vi "Apply Motor Transfer.vi"(10 "Right Motor":dbl, 11 "Left Motor":dbl) -> (2 "Right Motor Voltage":dbl, 3 "Left Motor Voltage":dbl)   [LabVIEW 2016]
uses:
  Globals/Motor Transfer.vi
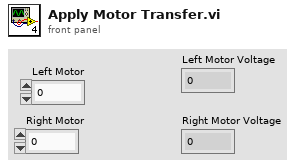
[diagram p1: front panel]
types:
  T1 = cluster{"Positive":cluster{"Slope":dbl, "Intercept":dbl}, "Negative":cluster{"Slope":dbl, "Intercept":dbl}}[]
  T2 = cluster{"Transfer[0]":cluster{"Positive":cluster{"Slope":dbl, "Intercept":dbl}, "Negative":cluster{"Slope":dbl, "Intercept":dbl}}, "Transfer[1]":cluster{"Positive":cluster{"Slope":dbl, "Intercept":dbl}, "Negative":cluster{"Slope":dbl, "Intercept":dbl}}}
  T3 = cluster{"Positive":cluster{"Slope":dbl, "Intercept":dbl}, "Negative":cluster{"Slope":dbl, "Intercept":dbl}}
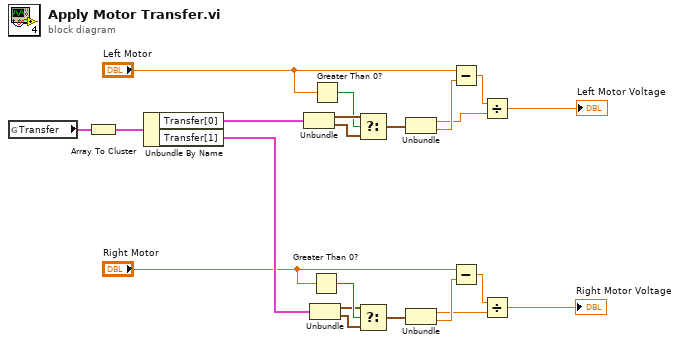
[diagram p0: block diagram]
diagram:
  n1 = global read "Motor Transfer.vi" "Transfer"() -> (w6:T1)
  n2 = Array To Cluster(array=w6) -> (cluster=w5:T2)
  n3 = Unbundle By Name(w5) -> ("Transfer[0]"=w4:T3, "Transfer[1]"=w3:T3)
  n4 = Unbundle(w4) -> ("Positive"=w21:cluster{"Slope":dbl, "Intercept":dbl}, "Negative"=w20:cluster{"Slope":dbl, "Intercept":dbl})
  n5 = Unbundle(w3) -> ("Positive"=w8:cluster{"Slope":dbl, "Intercept":dbl}, "Negative"=w7:cluster{"Slope":dbl, "Intercept":dbl})
  n6 = Greater Than 0?(x="Right Motor") -> (x > 0?=w13:bool)
  n7 = Greater Than 0?(x="Left Motor") -> (x > 0?=w19:bool)
  n8 = Select(t=w21, s=w19, f=w20) -> (s? t:f=w22:cluster{"Slope":dbl, "Intercept":dbl})
  n9 = Select(t=w8, s=w13, f=w7) -> (s? t:f=w14:cluster{"Slope":dbl, "Intercept":dbl})
  n10 = Unbundle(w22) -> ("Slope"=w16:dbl, "Intercept"=w18:dbl)
  n11 = Unbundle(w14) -> ("Slope"=w10:dbl, "Intercept"=w12:dbl)
  n12 = Subtract(x="Left Motor", y=w18) -> (x-y=w17:dbl)
  n13 = Subtract(x="Right Motor", y=w12) -> (x-y=w11:dbl)
  n14 = Divide(x=w17, y=w16) -> (x/y=→"Left Motor Voltage":dbl)
  n15 = Divide(x=w11, y=w10) -> (x/y=→"Right Motor Voltage":dbl)
